vi "Add.vi"() -> ()   [LabVIEW 2024, in "VarCircularBuffer.Tests.Units.lvlib"]
uses:
  VarCircularBuffer.Tests.Units.lvlib
  VarCircularBuffer.lvclass/VarCircularBuffer.ctl
  IsFull.vi
  Flush.vi/9e5e380d-a9b6-4c49-a1d6-4829efd6953e.vi
  Flush.vi/9e5e380d-a9b6-4c49-a1d6-4829efd6953e.vi/83cdeaba-e1ff-493a-b62c-1f93efcfb5e6.vi
  <vilib>/addons/_JKI Toolkits/Caraya/classes/Assert/Assert True.vi
  <vilib>/addons/_JKI Toolkits/Caraya/classes/Assert/Assert.lvclass
  <vilib>/addons/_JKI Toolkits/Caraya/classes/Test/Test.lvclass
  VarCircularBuffer.lvclass
panel:
  in  "Expected":variant[](array[variant])=[variant(i32 1), variant(i32 2), variant(i32 3), variant(i32 4), variant(i32 5), variant(i32 6), variant(i32 7), variant(i32 8), variant(i32 9), variant(i32 10)]
  out "Flushed Buffer":variant[](array[variant])
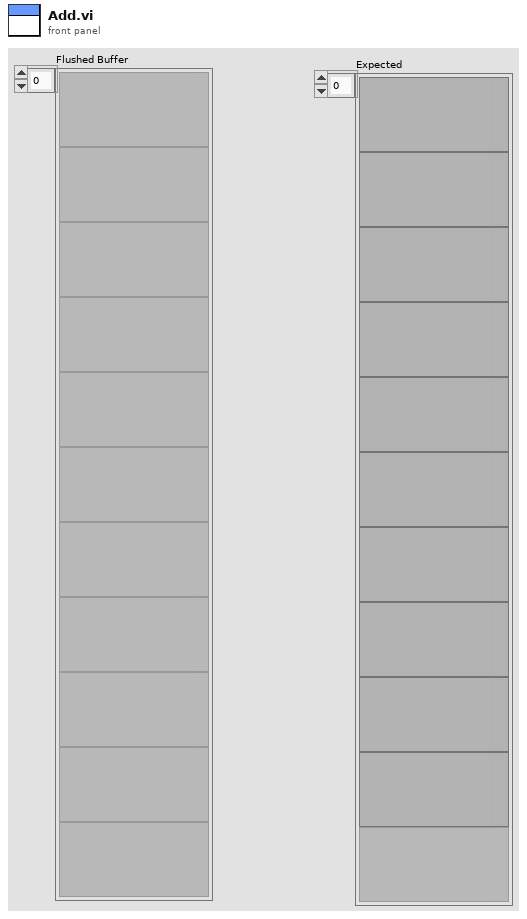
[diagram p1: front panel]
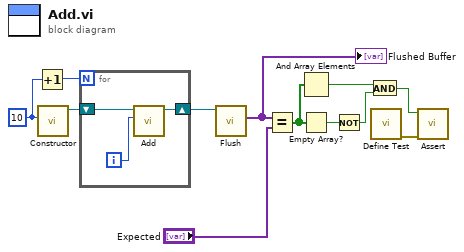
[diagram p0: block diagram]
diagram:
  w10 = u32 10 ("Capacity")
  n1 = Increment(x=w10) -> (x+1=w11:u32)
  n2 = call "Constructor.vi"("Capacity"=w10) -> ("TypedCircularBuffer out"=w12:refnum<class "VarCircularBuffer.lvclass">)  [unwired: 10 in]
  n3 = for {
    N: w11 -> [_]
    shift-right: [w14] -> w9
    shift-left: w12 -> [w15]
    i -> [w13]
    n4 = call "Add.vi"("Element"=w13, "TypedCircularBuffer in"=w15) -> ("TypedCircularBuffer out"=w14:refnum<class "VarCircularBuffer.lvclass">)  [unwired: 7 in, 2 out]
  }
  n5 = call "Flush.vi"("TypedCircularBuffer in"=w9) -> ("Flushed Buffer"=w8:variant[])  [unwired: 9 in, 1 out]
  "Flushed Buffer" <- w8
  n6 = Equal?(x=w8, y="Expected") -> (x = y?=w4:bool[])
  n7 = And Array Elements(Boolean array=w4) -> (logical AND=w7:bool)
  n8 = Empty Array?(array=w4) -> (empty?=w6:bool)
  n9 = Not(x=w6) -> (.not. x?=w5:bool)
  n10 = And(x=w7, y=w5) -> (x .and. y?=w3:bool)
  n11 = call <vilib>:"Define Test.vi"() -> ("error out"=w2:errorcluster)  [unwired: 10 in, 1 out]
  n12 = call-poly <vilib>:"Assert.vi"("error in (no error)"=w2, "True?"=w3) -> ()  [unwired: 8 in, 2 out]
